vi "Grid Image.vi"(11 "image data":T1) -> (1 "Vertical Grid Size":i32, 2 "Horizontal Grid Size":i32, 3 "Grid of 2D Pixel Arrays":u32[][][](array[colorbox]), 4 "Horizontal Grid Divisions":i32=10, 6 "Vertical Grid Divisions":i32=10)   [LabVIEW 2014, in "Histogram Grid Comparison.lvclass"]
uses:
  Histogram Grid Comparison.lvclass
  Image Comparison/Image Comparison.lvclass
  <vilib>/picture/picture.llb/imagedata.ctl
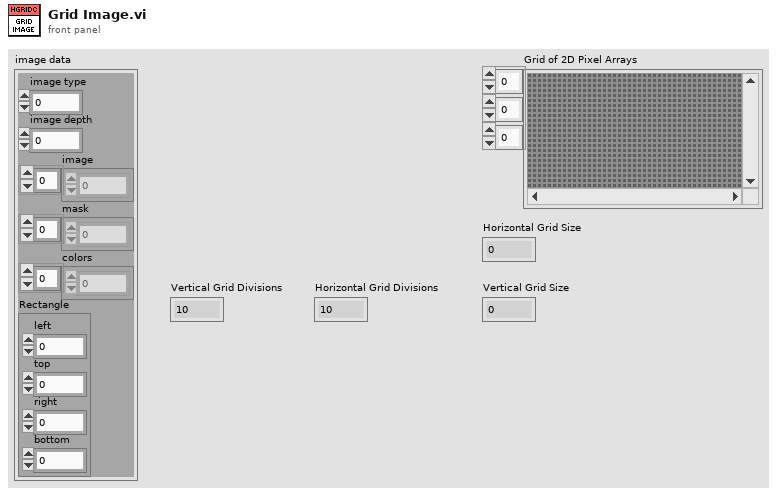
[diagram p1: front panel]
types:
  T1 = typedef "imagedata.ctl" = cluster{"image type":i32, "image depth":i32, "image":u8[], "mask":u8[], "colors":u32[], "Rectangle":cluster{"left":i16, "top":i16, "right":i16, "bottom":i16}}
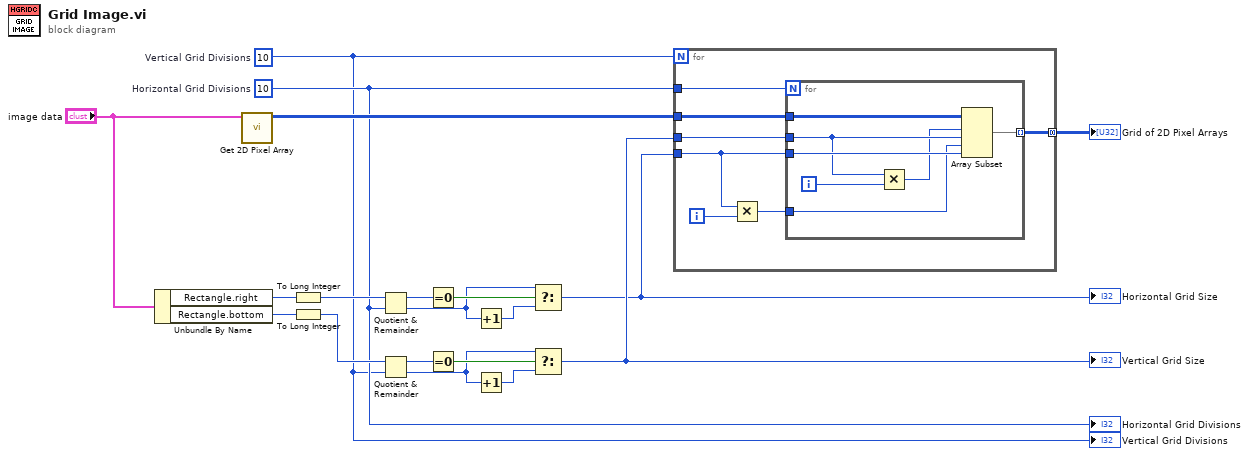
[diagram p0: block diagram]
diagram:
  w1 = 10  # Vertical Grid Divisions
  w2 = 10  # Horizontal Grid Divisions
  n1 = Unbundle By Name("image data") -> ("Rectangle.right"=w17:i16, "Rectangle.bottom"=w18:i16)
  n2 = call "Get 2D Pixel Array.vi"("image data"="image data") -> ("2D Pixel Array"=w6:u32[][])  [unwired: 10 in]
  n3 = To Long Integer(number=w17) -> (32bit integer=w16:i32)
  n4 = To Long Integer(number=w18) -> (32bit integer=w15:i32)
  n5 = Quotient & Remainder(x=w16, y=w2) -> (x-y*floor(x/y)=w14:i32, floor(x/y)=w12:i32)
  n6 = Quotient & Remainder(x=w15, y=w1) -> (x-y*floor(x/y)=w8:i32, floor(x/y)=w7:i32)
  n7 = Equal To 0?(x=w14) -> (x = 0?=w13:bool)
  n8 = Equal To 0?(x=w8) -> (x = 0?=w9:bool)
  n9 = Increment(x=w12) -> (x+1=w11:i32)
  n10 = Increment(x=w7) -> (x+1=w10:i32)
  n11 = Select(t=w12, s=w13, f=w11) -> (s? t:f=w4:i32)
  "Horizontal Grid Size" <- w4
  n12 = Select(t=w7, s=w9, f=w10) -> (s? t:f=w5:i32)
  "Vertical Grid Size" <- w5
  n13 = for {
    N: w1 -> [_]
    tunnel: w6 -> [w26]
    tunnel: w5 -> [w25]
    tunnel: w4 -> [w23]
    tunnel: [w21] -> w3 mode=concatenating
    tunnel: w2 -> [w20]
    i -> [w24]
    n14 = Multiply(x=w23, y=w24) -> (x*y=w22:i32)
    n15 = for {
      N: w20 -> [_]
      tunnel: w26 -> [w32]
      tunnel: w25 -> [w30]
      tunnel: w23 -> [w33]
      tunnel: w22 -> [w28]
      tunnel: [w27] -> w21 mode=indexing
      i -> [w31]
      n16 = Multiply(x=w30, y=w31) -> (x*y=w29:i32)
      n17 = Array Subset(array=w32, index (row)=w29, length (row)=w30, index (col)=w28, length (col)=w33) -> (w27:u32[][])
    }
  }
  "Grid of 2D Pixel Arrays" <- w3
  "Vertical Grid Divisions" <- w1
  "Horizontal Grid Divisions" <- w2
